vi "test_dragon_file--list_vipm_dependencies_(packages).vi"(8 "error in (no error)":errorcluster) -> (0 "error out":errorcluster)   [LabVIEW 2020]
uses:
  c4136637-9e6b-4610-ba28-79e7dff09705.vi
  c4136637-9e6b-4610-ba28-79e7dff09705.vi/05157253-4ade-4b75-9902-c642c5dd4762.vi
  c4136637-9e6b-4610-ba28-79e7dff09705.vi/543db544-a529-4041-9332-0fe0cbee0c9f.vi
  toml/read_subtable_key_string.vi
  toml/toml.lvclass
  <vilib>/addons/_JKI Toolkits/Caraya/classes/Assert/Assert.lvclass
  <vilib>/addons/_JKI Toolkits/Caraya/classes/Test/Test.lvclass
panel:
  out "package-versions":string[](array[string])
  out "package-names":string[](array[string])
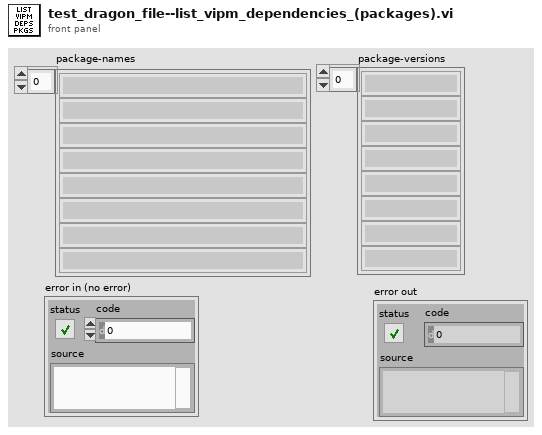
[diagram p1: front panel]
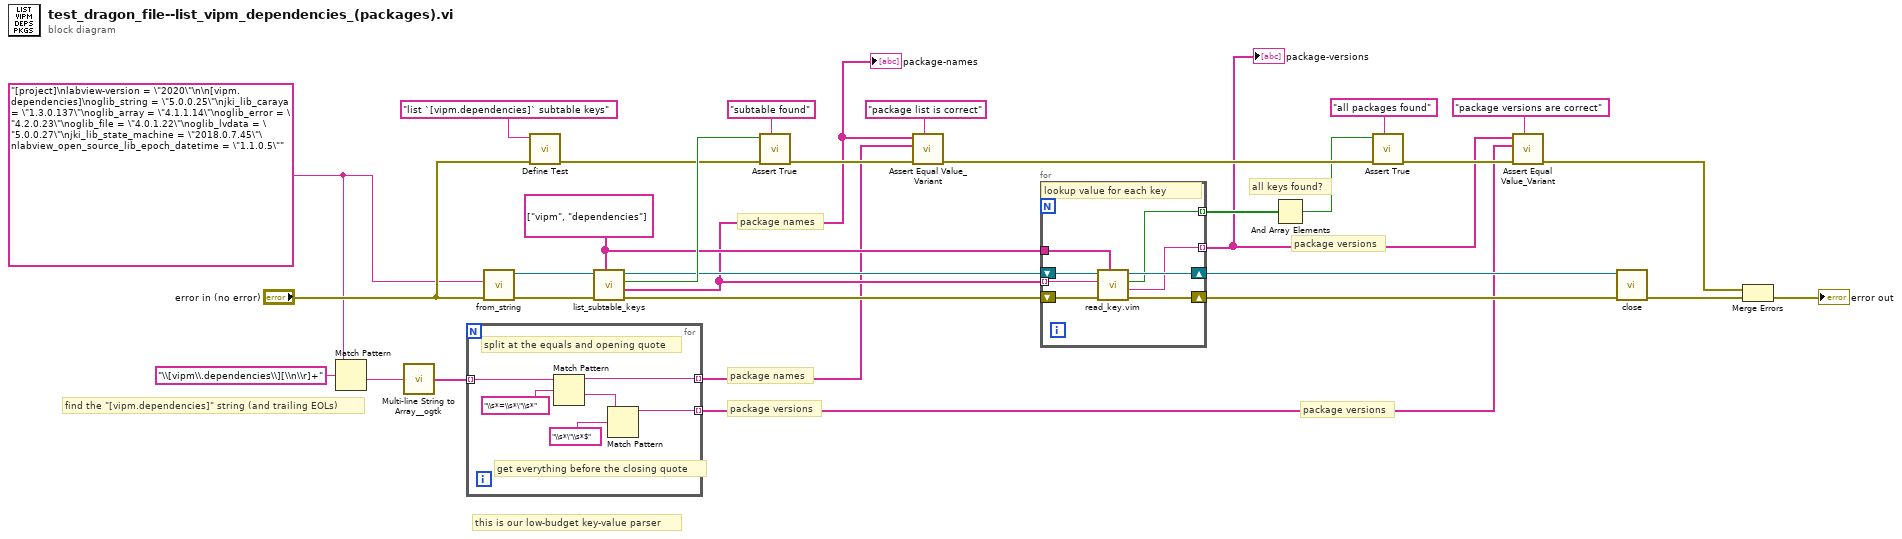
[diagram p0: block diagram]
diagram:
  w19 = string[] ["vipm", "dependencies"]
  w4 = "[project]\nlabview-version = \"2020\"\n\n[vipm.dependencies]\noglib_string = \"5.0.0.25\"\njki_lib_caraya = \"1.3.0.137\"\noglib_array = \"4.1.1.14\"\noglib_error = \"4.2.0.23\"\noglib_file = \"4.0.1.22\"\noglib_lvdata = \"5.0.0.27\"\njki_lib_state_machine = \"2018.0.7.45\"\nlabview_open_source_lib_epoch_datetime = \"1.1.0.5\"" ("toml_string in")
  # "package versions"
  # "this is our low-budget key-value parser"
  # "find the \"[vipm.dependencies]\" string (and trailing EOLs)"
  # "all keys found?"
  # "package versions"
  # "package versions"
  # "package names"
  # "package names"
  n1 = Match Pattern(string=w4, regular expression="\\[vipm\\.dependencies\\][\\n\\r]+") -> (after substring=w3:string)  [unwired: 1 in, 3 out]
  n2 = call <userlib>:"Multi-line String to Array__ogtk.vi"("string"=w3) -> ("lines"=w10:string[])
  n3 = for {
    tunnel: w10 -> [w37] mode=indexing
    tunnel: [w35] -> w9 mode=indexing
    tunnel: [w32] -> w1 mode=indexing
    # "get everything before the closing quote"
    # "split at the equals and opening quote"
    n4 = Match Pattern(string=w37, regular expression="\\s*=\\s*\"\\s*") -> (before substring=w35:string, after substring=w34:string)  [unwired: 1 in, 2 out]
    n5 = Match Pattern(string=w34, regular expression="\\s*\"\\s*$") -> (before substring=w32:string)  [unwired: 1 in, 3 out]
  }
  n6 = call "from_string.vi"("error in (no error)"="error in (no error)", "toml"=w4) -> ("error out"=w27:errorcluster, "toml out"=w28:refnum<class "toml.lvclass">)  [unwired: 8 in]
  n7 = call <vilib>:"Define Test.vi"("error in (no error)"="error in (no error)", "Label (VI Title)"="list `[vipm.dependencies]` subtable keys") -> ("error out"=w22:errorcluster)  [unwired: 9 in]
  n8 = call "list_subtable_keys.vi"("subtables"=w19, "error in (no error)"=w27, "toml in"=w28) -> ("error out"=w18:errorcluster, "keys"=w15:string[], "subtable found?"=w24:bool, "toml out"=w20:refnum<class "toml.lvclass">)  [unwired: 5 in]
  "package-names" <- w15
  n9 = call <vilib>:"Assert True.vi"("Label"="subtable found", "error in (no error)"=w22, "True?"=w24) -> ("error out"=w21:errorcluster)  [unwired: 8 in]
  n10 = call <vilib>:"Assert Equal Value_Variant.vi"("Label"="package list is correct", "error in (no error)"=w21, "Y"=w9, "X"=w15) -> ("error out"=w12:errorcluster)  [unwired: 7 in]
  n11 = for {
    tunnel: w19 -> [w44]
    shift-right: [w43] -> w16
    shift-left: w20 -> [w45]
    shift-right: [w41] -> w17
    shift-left: w18 -> [w42]
    tunnel: w15 -> [w40] mode=indexing
    tunnel: [w39] -> w14 mode=indexing
    tunnel: [w38] -> w2 mode=indexing
    # "lookup value for each key"
    n12 = call "read_key.vim"("table"=w44, "error in (no error)"=w42, "key"=w40, "toml in"=w45) -> ("error out"=w41:errorcluster, "value"=w38:string, "found?"=w39:bool, "toml out"=w43:refnum<class "toml.lvclass">)  [unwired: 4 in]
  }
  "package-versions" <- w2
  n13 = And Array Elements(Boolean array=w14) -> (logical AND=w11:bool)
  n14 = call <vilib>:"Assert True.vi"("Label"="all packages found", "error in (no error)"=w12, "True?"=w11) -> ("error out"=w8:errorcluster)  [unwired: 8 in]
  n15 = call <vilib>:"Assert Equal Value_Variant.vi"("Label"="package versions are correct", "error in (no error)"=w8, "Y"=w1, "X"=w2) -> ("error out"=w7:errorcluster)  [unwired: 7 in]
  n16 = call "close.vi"("error in (no error)"=w17, "toml in"=w16) -> ("error out"=w26:errorcluster)  [unwired: 9 in]
  n17 = Merge Errors(w7, w26) -> (→"error out":errorcluster)
